vi "Globals.vi"() -> ()   [LabVIEW 2014]
panel:
  out "Encoders":T1(array[cluster])
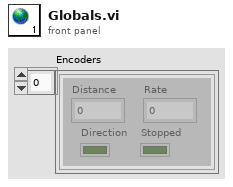
[diagram p1: front panel]
types:
  T1 = cluster{"Distance":dbl, "Rate":dbl, "Direction":bool, "Stopped":bool}[]
diagram:
